vi "Water Valves.vi"(1 "Water Valve Input 3":T2={"Fine Water Adjust (valve)"=100.0, "Accept Autotune Water Valve"=FALSE, "Fine slide in P"=refnum, "file for water valve"=path "", "autotune? water valve"=FALSE, "PID gains in water valve"={"proportional gain (Kc)"=0.0, "integral time (Ti, min)"=0.0, "derivative time (Td, min)"=0.0}} {"Fine Water Adjust (valve)" min=0.0 max=100.0 step=1.0 scale=0.0..100.0}, 4 "Condensing Press Threshold":dbl=10.0 format="%#_13g", 5 "Water Valve Input 2":T2={"Fine Water Adjust (valve)"=100.0, "Accept Autotune Water Valve"=FALSE, "Fine slide in P"=refnum, "file for water valve"=path "", "autotune? water valve"=FALSE, "PID gains in water valve"={"proportional gain (Kc)"=0.0, "integral time (Ti, min)"=0.0, "derivative time (Td, min)"=0.0}} {"Fine Water Adjust (valve)" min=0.0 max=100.0 step=1.0 scale=0.0..100.0}, 6 "Current Pcond":dbl, 7 "Desired Pcond":dbl, 8 "Water Pump Input":T4={"Coarse Water Adjust (pump)"=100.0, "Accept Autotune Water Pump"=FALSE, "Coarse slide in P"=refnum, "file for water pump"=path "", "autotune? water pump"=FALSE, "PID gains in water pump"={"proportional gain (Kc)"=0.0, "integral time (Ti, min)"=0.0, "derivative time (Td, min)"=0.0}} {"Coarse Water Adjust (pump)" min=0.0 max=100.0 step=1.0 scale=0.0..100.0}, 9 "Reinitialize Controller":bool, 10 "Controller Toggle P 2":bool, 11 "Water Valve Input":T2={"Fine Water Adjust (valve)"=100.0, "Accept Autotune Water Valve"=FALSE, "Fine slide in P"=refnum, "file for water valve"=path "", "autotune? water valve"=FALSE, "PID gains in water valve"={"proportional gain (Kc)"=0.0, "integral time (Ti, min)"=0.0, "derivative time (Td, min)"=0.0}} {"Fine Water Adjust (valve)" min=0.0 max=100.0 step=1.0 scale=0.0..100.0}) -> (0 "output cluster":T1, 2 "output cluster 2":T1, 3 "Water Control Out":T3)   [LabVIEW 2017]
doc: "Control logic for all controllers on water line. Thresholding procedure that determines which controller should be operating based on current process variable. Passes the chosen controller to the PID vi's"
panel:
  out "output to valve 2":dbl
  in  "Controller Toggle P 4":bool=TRUE
  in  "Reinitialize Controller  3":bool
  out "output to valve":dbl
  in  "Controller Toggle P 3":bool=TRUE
  in  "Reinitialize Controller  2":bool
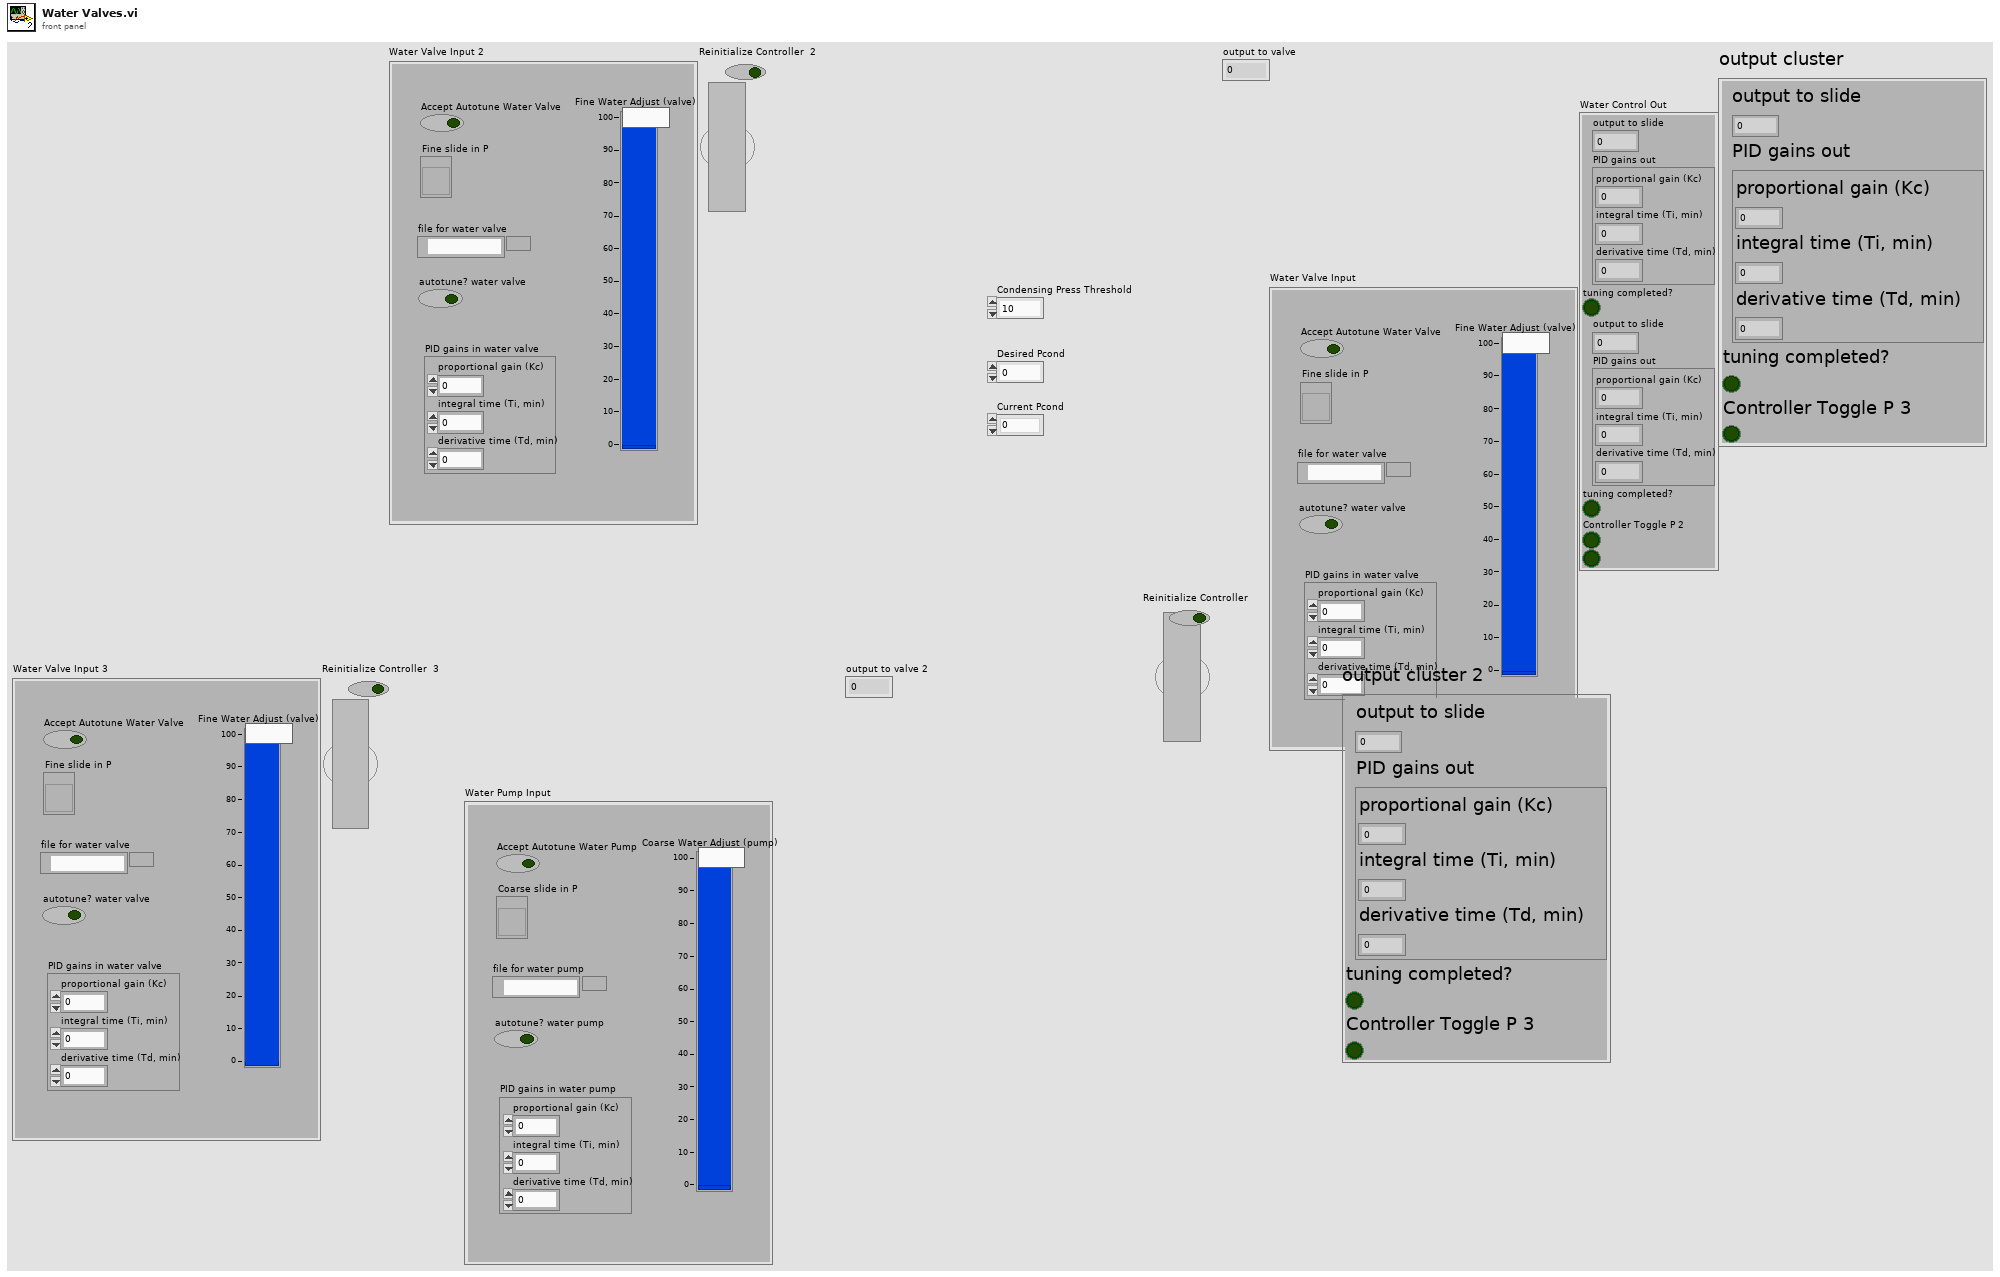
[diagram p1: front panel]
types:
  T1 = cluster{"output to slide":dbl, "PID gains out":cluster{"proportional gain (Kc)":dbl, "integral time (Ti, min)":dbl, "derivative time (Td, min)":dbl}, "tuning completed?":bool, "Controller Toggle P 3":bool}
  T2 = cluster{"Fine Water Adjust (valve)":dbl, "Accept Autotune Water Valve":bool, "Fine slide in P":refnum<vi>, "file for water valve":path, "autotune? water valve":bool, "PID gains in water valve":cluster{"proportional gain (Kc)":dbl, "integral time (Ti, min)":dbl, "derivative time (Td, min)":dbl}}
  T3 = cluster{"output to slide":dbl, "PID gains out":cluster{"proportional gain (Kc)":dbl, "integral time (Ti, min)":dbl, "derivative time (Td, min)":dbl}, "tuning completed?":bool, "output to slide":dbl, "PID gains out":cluster{"proportional gain (Kc)":dbl, "integral time (Ti, min)":dbl, "derivative time (Td, min)":dbl}, "tuning completed?":bool, "Controller Toggle P 2":bool, bool}
  T4 = cluster{"Coarse Water Adjust (pump)":dbl, "Accept Autotune Water Pump":bool, "Coarse slide in P":refnum<vi>, "file for water pump":path, "autotune? water pump":bool, "PID gains in water pump":cluster{"proportional gain (Kc)":dbl, "integral time (Ti, min)":dbl, "derivative time (Td, min)":dbl}}
  T5 = cluster{"proportional gain (Kc)":dbl, "integral time (Ti, min)":dbl, "derivative time (Td, min)":dbl}
  T6 = enum8{"Enabled", "Disabled", "Disabled and Grayed Out"}
  T7 = cluster{"output to slide":dbl, "PID gains out":cluster{"proportional gain (Kc)":dbl, "integral time (Ti, min)":dbl, "derivative time (Td, min)":dbl}, "tuning completed?":bool, "Controller Toggle P 4":bool}
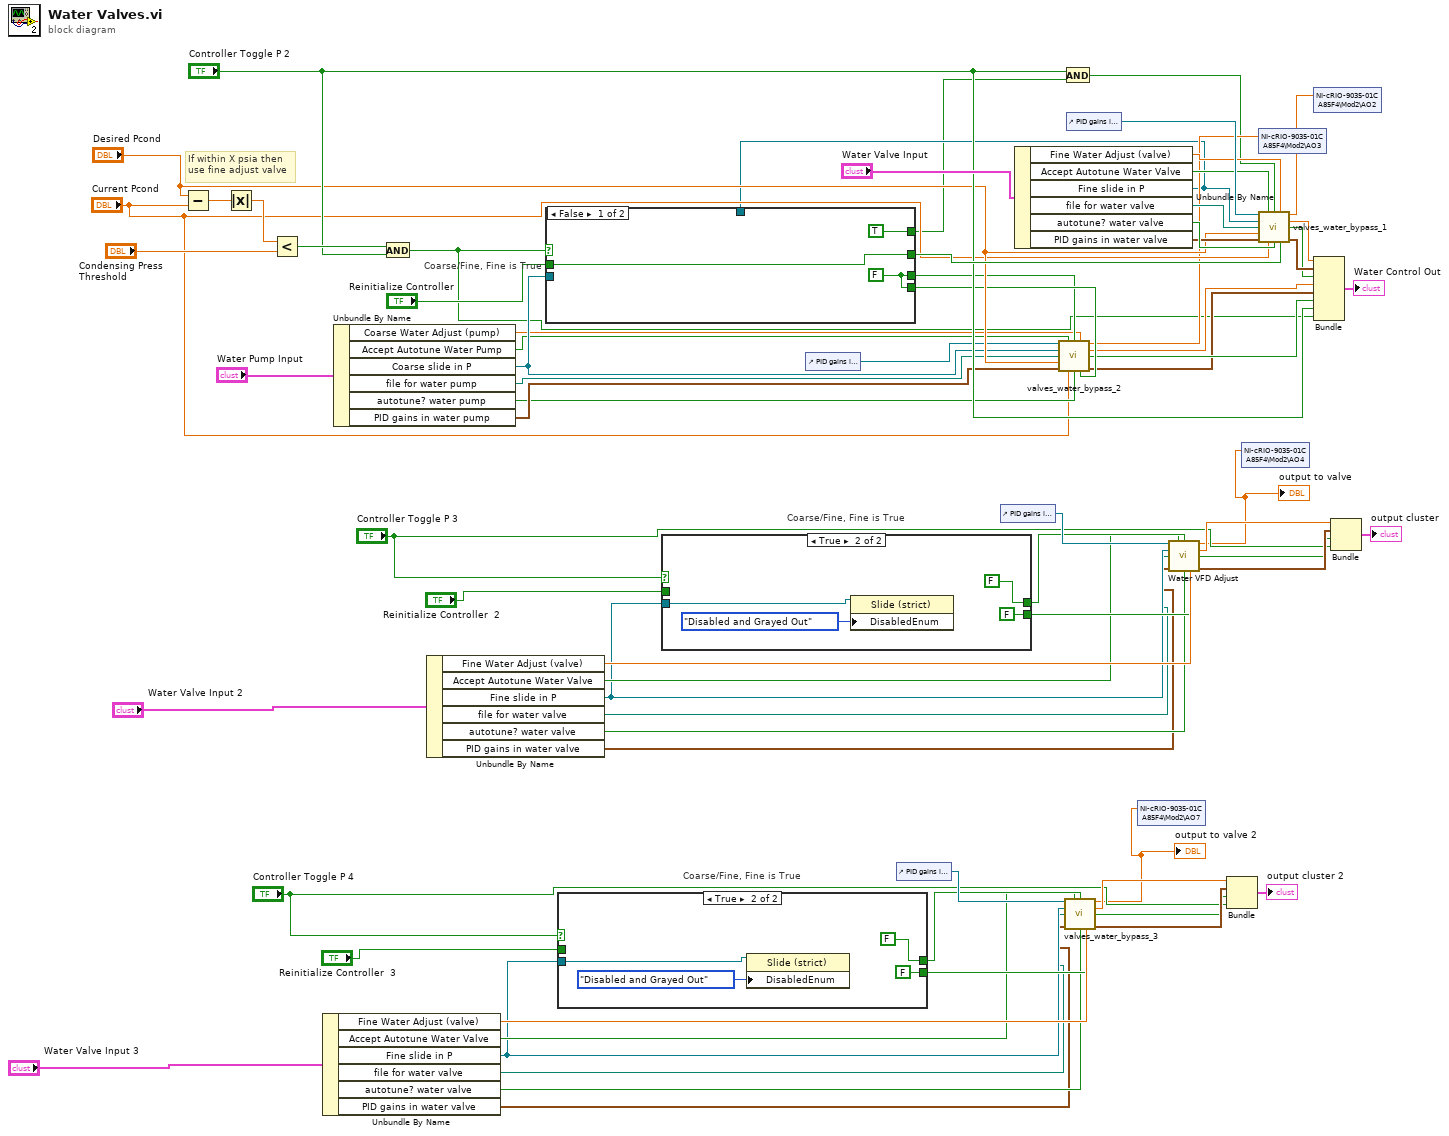
[diagram p0: block diagram]
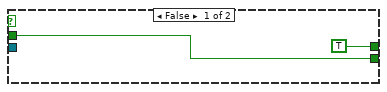
[diagram p2: hidden frame]
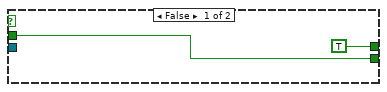
[diagram p3: hidden frame]
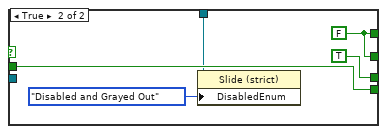
[diagram p4: hidden frame]
diagram:
  # "If within X psia then\nuse fine adjust valve"
  n1 = Subtract(x="Desired Pcond", y="Current Pcond") -> (x-y=w59:dbl)
  n2 = Absolute Value(x=w59) -> (abs(x)=w58:dbl)
  n3 = Less?(x=w58, y="Condensing Press Threshold") -> (x < y?=w56:bool)
  n4 = Unbundle By Name("Water Valve Input 3") -> ("Fine Water Adjust (valve)"=w18:dbl, "Accept Autotune Water Valve"=w14:bool, "Fine slide in P"=w13:refnum<vi>, "file for water valve"=w12:path, "autotune? water valve"=w11:bool, "PID gains in water valve"=w10:T5)
  n5 = Unbundle By Name("Water Pump Input") -> ("Coarse Water Adjust (pump)"=w44:dbl, "Accept Autotune Water Pump"=w46:bool, "Coarse slide in P"=w51:refnum<vi>, "file for water pump"=w52:path, "autotune? water pump"=w48:bool, "PID gains in water pump"=w54:T5)
  n6 = And(x=w56, y="Controller Toggle P 2") -> (x .and. y?=w38:bool)
  n7 = Unbundle By Name("Water Valve Input 2") -> ("Fine Water Adjust (valve)"=w35:dbl, "Accept Autotune Water Valve"=w31:bool, "Fine slide in P"=w30:refnum<vi>, "file for water valve"=w29:path, "autotune? water valve"=w28:bool, "PID gains in water valve"=w27:T5)
  n8 = case "Coarse/Fine, Fine is True" shown="True" "Controller Toggle P 4" {
    tunnel: "Reinitialize Controller  3" -> [w74 _]
    tunnel: [w74 FALSE] -> w16
    tunnel: [TRUE FALSE] -> w15
    tunnel: w13 -> [_ w77]
    frame False {
    }
    frame True {
      n9 = property on="Property Node" class="Slide (strict)"(reference=w77, "DisabledEnum"=T6."Disabled and Grayed Out" ("Disabled")) -> ()  [unwired: 1 in, 2 out]
    }
  }
  n10 = case "Coarse/Fine, Fine is True" shown="True" "Controller Toggle P 3" {
    tunnel: "Reinitialize Controller  2" -> [w80 _]
    tunnel: [w80 FALSE] -> w33
    tunnel: [TRUE FALSE] -> w32
    tunnel: w30 -> [_ w83]
    frame False {
    }
    frame True {
      n11 = property on="Property Node" class="Slide (strict)"(reference=w83, "DisabledEnum"=T6."Disabled and Grayed Out" ("Disabled")) -> ()  [unwired: 1 in, 2 out]
    }
  }
  n12 = control-ref of="PID gains in water pump"() -> (w50:refnum<vi>)
  n13 = control-ref of="PID gains in water valve"() -> (w17:refnum<vi>)
  n14 = control-ref of="PID gains in water valve"() -> (w34:refnum<vi>)
  n15 = Unbundle By Name("Water Valve Input") -> ("Fine Water Adjust (valve)"=w65:dbl, "Accept Autotune Water Valve"=w64:bool, "Fine slide in P"=w39:refnum<vi>, "file for water valve"=w63:path, "autotune? water valve"=w62:bool, "PID gains in water valve"=w61:T5)
  n16 = case "Coarse/Fine, Fine is True" shown="False" w38 {
    tunnel: [TRUE w89] -> w2
    tunnel: "Reinitialize Controller" -> [w87 w93]
    tunnel: [w87 w89] -> w71
    tunnel: [w86 w93] -> w49
    tunnel: [w86 TRUE] -> w45
    tunnel: w51 -> [_ _]
    tunnel: w39 -> [_ w91]
    frame False {
      w86 = FALSE
    }
    frame True {
      w89 = FALSE
      n17 = property on="Property Node" class="Slide (strict)"(reference=w91, "DisabledEnum"=T6."Disabled and Grayed Out" ("Disabled")) -> ()  [unwired: 1 in, 2 out]
    }
  }
  n18 = call "valves_water_bypass_2.vi"("PID Gains Cluster Ref"=w50, "Accept Autotune"=w46, "Controller Toggle (Manual Mode)"=w45, "Valve Manual Adjust"=w44, "Slide Refnum in"=w51, "file (use dialog)"=w52, "Desired Setpoint"="Desired Pcond", "PID gains"=w54, "Current Process Variable Value"="Current Pcond", "autotune? (F)"=w48, "Reinitialize Controller"=w49) -> ("output to valve"=w43:dbl, "output to slide"=w42:dbl, "tuning completed?"=w41:bool, "PID gains out"=w40:T5)  [unwired: 1 out]
  n19 = And(x="Controller Toggle P 2", y=w2) -> (x .and. y?=w1:bool)
  n20 = call "valves_water_bypass_3.vi"("PID Gains Cluster Ref"=w17, "Accept Autotune"=w14, "Controller Toggle (Manual Mode)"=w15, "Valve Manual Adjust"=w18, "Slide Refnum in"=w13, "file (use dialog)"=w12, "PID gains"=w10, "autotune? (F)"=w11, "Reinitialize Controller"=w16) -> ("output to valve"=w3:dbl, "output to slide"=w9:dbl, "tuning completed?"=w7:bool, "PID gains out"=w8:T5)  [unwired: 2 in, 1 out]
  "output to valve 2" <- w3
  n21 = control-ref of="PID gains in water valve"() -> (w70:refnum<vi>)
  n22 = shared-variable "NI-cRIO-9035-01CA85F4\\Mod2\\AO7"(w3) -> ()  [unwired: 1 in, 1 out]
  n23 = call "Water VFD Adjust.vi"("PID Gains Cluster Ref"=w34, "Accept Autotune"=w31, "Controller Toggle (Manual Mode)"=w32, "Valve Manual Adjust"=w35, "Slide Refnum in"=w30, "file (use dialog)"=w29, "PID gains"=w27, "autotune? (F)"=w28, "Reinitialize Controller"=w33) -> ("output to valve"=w20:dbl, "output to slide"=w26:dbl, "tuning completed?"=w24:bool, "PID gains out"=w25:T5)  [unwired: 2 in, 1 out]
  "output to valve" <- w20
  n24 = Bundle("output to slide"=w9, "PID gains out"=w8, "tuning completed?"=w7, "Controller Toggle P 4"="Controller Toggle P 4") -> (→"output cluster 2":T7)  [unwired: 1 in]
  n25 = shared-variable "NI-cRIO-9035-01CA85F4\\Mod2\\AO4"(w20) -> ()  [unwired: 1 in, 1 out]
  n26 = shared-variable "NI-cRIO-9035-01CA85F4\\Mod2\\AO3"(w43) -> ()  [unwired: 1 in, 1 out]
  n27 = call "valves_water_bypass_1.vi"("PID Gains Cluster Ref"=w70, "Accept Autotune"=w64, "Controller Toggle (Manual Mode)"=w1, "Valve Manual Adjust"=w65, "Slide Refnum in"=w39, "file (use dialog)"=w63, "Desired Setpoint"="Desired Pcond", "PID gains"=w61, "Current Process Variable Value"="Current Pcond", "autotune? (F)"=w62, "Reinitialize Controller"=w71) -> ("output to valve"=w66:dbl, "output to slide"=w69:dbl, "tuning completed?"=w67:bool, "PID gains out"=w68:T5)  [unwired: 1 out]
  n28 = shared-variable "NI-cRIO-9035-01CA85F4\\Mod2\\AO2"(w66) -> ()  [unwired: 1 in, 1 out]
  n29 = Bundle("output to slide"=w69, "PID gains out"=w68, "tuning completed?"=w67, "output to slide"=w42, "PID gains out"=w40, "tuning completed?"=w41, "Controller Toggle P 2"="Controller Toggle P 2", w38) -> (→"Water Control Out":T3)  [unwired: 1 in]
  n30 = Bundle("output to slide"=w26, "PID gains out"=w25, "tuning completed?"=w24, "Controller Toggle P 3"="Controller Toggle P 3") -> (→"output cluster":T1)  [unwired: 1 in]
